vi "UDP_Server.vi"() -> ()   [LabVIEW 2020]
uses:
  <vilib>/ErrorRing/Error Ring.xnode
panel:
  in  "String":string
  in  "Puerto Destino":u16
  out "data out":string
  in  "stop":bool
  # "Server UDP Numero 1"
  # "Cliente UDP Numero 2"
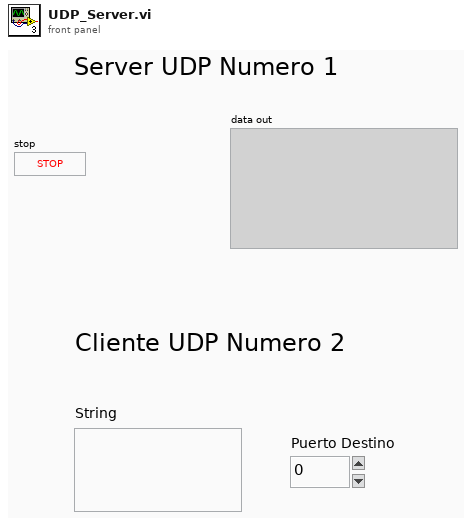
[diagram p1: front panel]
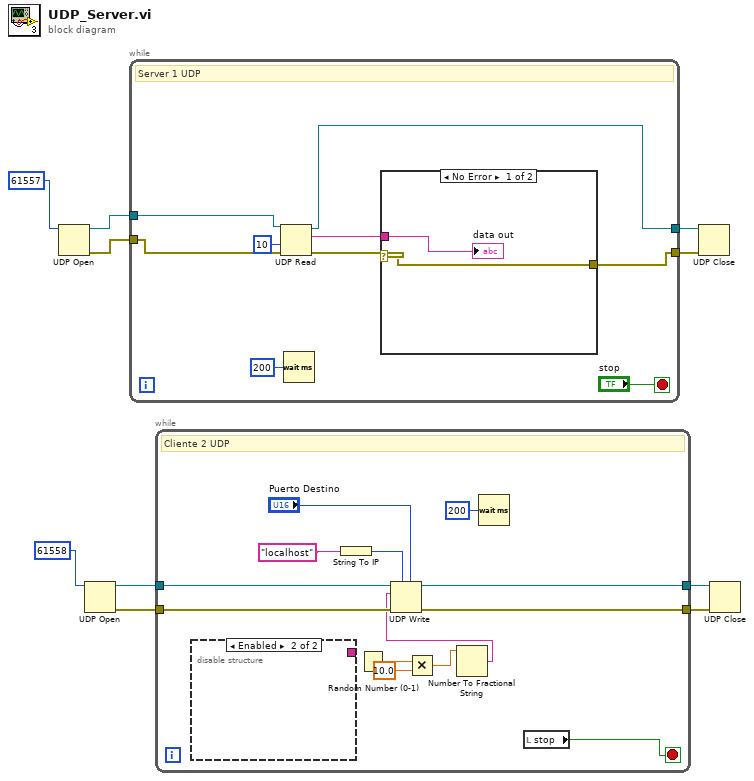
[diagram p0: block diagram]
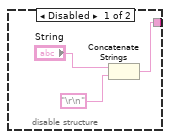
[diagram p2: hidden frame]
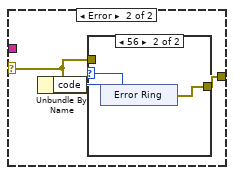
[diagram p3: hidden frame]
diagram:
  n1 = UDP Open(11:u16 61557 ("port")) -> (port=w9:refnum<k16>, 0:w10:errorcluster)  [unwired: 4 in, 1 out]
  n2 = UDP Open(11:u16 61558 ("port")) -> (port=w2:refnum<k16>, 0:w5:errorcluster)  [unwired: 4 in, 1 out]
  n3 = while {
    tunnel: w10 -> [w17]
    tunnel: w9 -> [w18]
    tunnel: [w14] -> w7
    tunnel: [w12] -> w6
    stop <- "stop" stop-if-true
    # "Server 1 UDP"
    n4 = UDP Read(connection ID=w18, timeout ms (25000)=10, 8:w17) -> (data out=w13:string, error out=w15:errorcluster, 3:w14:refnum<k16>)  [unwired: 1 in, 2 out]
    n5 = Wait (ms)(milliseconds to wait=u32 200) -> ()  [unwired: 1 out]
    n6 = case shown="No Error" w15 {
      selector: w15 -> [w20 w22]
      tunnel: w13 -> [w21 _]
      tunnel: [w20 w23] -> w12
      frame No Error {
        "data out" <- w21
      }
      frame Error {
        n7 = Unbundle By Name(w22) -> ("code"=w24:i32)
        n8 = case shown="56" w24 {
          tunnel: [w25 w26] -> w23
          tunnel: w22 -> [w25 _]
          frame 0, Default {
          }
          frame 56 {
            n9 = xnode "Error Ring"() -> ("error out"=w26:errorcluster)
          }
        }
      }
    }
  }
  n10 = while {
    tunnel: w5 -> [w40]
    tunnel: [w39] -> w4
    tunnel: [w38] -> w3
    tunnel: w2 -> [w37]
    stop <- w33 stop-if-true
    # "Cliente 2 UDP"
    n11 = disable-structure shown="Enabled" {
      disable-tunnel: [w41 _] -> _
      frame Disabled {
        n12 = Concatenate Strings("String", "\r\n") -> (w41:string)
      }
      frame Enabled {
      }
    }
    n13 = String To IP(1:"localhost" ("name")) -> (0:w36:u32)
    n14 = Random Number (0-1)() -> (number: 0 to 1=w32:dbl)
    n15 = Multiply(x=w32, y=10.0) -> (x*y=w30:dbl)
    n16 = Number To Fractional String(number=w30) -> (F-format string=w29:string)  [unwired: 3 in]
    n17 = UDP Write(address=w36, port or service name="Puerto Destino", connection ID=w37, data in=w29, 8:w40) -> (error out=w39:errorcluster, 3:w38:refnum<k16>)  [unwired: 1 in]
    n18 = Wait (ms)(milliseconds to wait=u32 200) -> ()  [unwired: 1 out]
    n19 = local read "stop"() -> (w33:bool)
  }
  n20 = UDP Close(connection ID=w7, 8:w6) -> ()  [unwired: 2 out]
  n21 = UDP Close(connection ID=w3, 8:w4) -> ()  [unwired: 2 out]
